vi "SETMotorOFF.vi"(8 "error in":errorcluster, 11 "PicomotorController in":refnum<class "PicomotorController.lvclass">) -> (0 "error out":errorcluster, 3 "PicomotorController out":refnum<class "PicomotorController.lvclass">)   [LabVIEW 2020, in "PicomotorController.lvclass"]
uses:
  PicomotorController.lvclass
  MCL Cmd Cluster.ctl
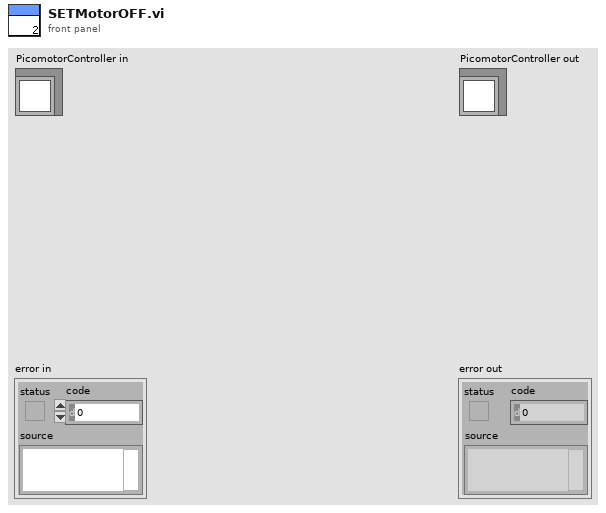
[diagram p1: front panel]
types:
  T1 = typedef "MCL Cmd Cluster.ctl" = cluster{"MCL Cmd":enum16{"User....", "DEF", "DIAG", "INI", "LOCK", "UNLOCK", "MAP", "SAV", "VER", "ACC", "CHL", "FOR", "GO", "HAL", "MOF", "MON", "MPV", "POS", "REL", "REV", "STA", "STO", "TYP", "VEL", "ABS", "SER", "NOS", "DRT", "FLI", "RLI", "FIN", "RIN", "AIN", "IN", "JOF", "JON", "OUT", "RES FINE", "RES COARSE", "02 (HEX)", "PWM", "CNT", "TMR", "HOSTNAME", "IPADDR", "IPMODE", "NETMASK", "GATEWAY", "DNSSRVR", "PASSWD", "ECHO", "MACADDR"}, "User Cmd/Numeric Argu":string, "Query/Set":enum16{"Query", "Set"}}
  T2 = typedef "VISA & TCPIP Control.ctl" = cluster{"Resource Name":refnum<visa-resource-name>, "Init VISA":bool, "Close VISA":bool, "VISA or TCP/IP":bool, "IP Address/Hostname":string}
  T3 = typedef "Pico Parameters.ctl" = cluster{"Pico Type":enum16{"Open-Loop Pico", "Close-Loop Pico", "Pico Ultra"}, "Acceleration (steps/sec^2)":string, "Velocity ( Hz)":string, "Driver":string, "Motor":string, "Channel":string, "Process Step":string}
  T4 = typedef "Error.ctl" = errorcluster
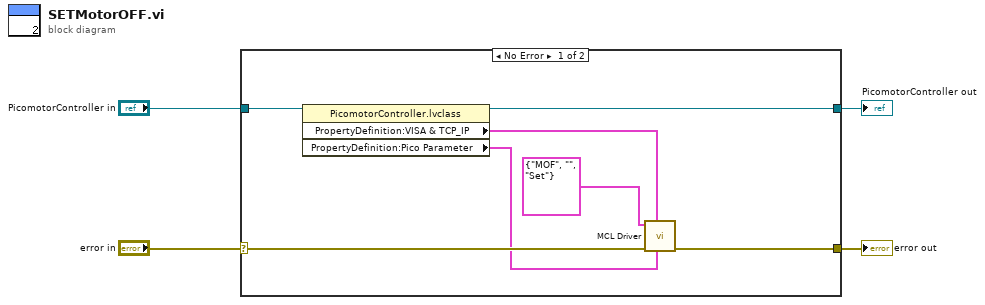
[diagram p0: block diagram]
diagram:
  n1 = case shown="No Error" "error in" {
    selector: "error in" -> [w7 w13]
    tunnel: [w6 w13] -> w3
    tunnel: [w8 w12] -> w1
    tunnel: "PicomotorController in" -> [w9 w12]
    frame No Error {
      n2 = property class="PicomotorController.lvclass"(reference=w9) -> (reference out=w8:refnum<class "PicomotorController.lvclass">, "PropertyDefinition:VISA & TCP_IP"=w11:T2, "PropertyDefinition:Pico Parameter"=w5:T3)  [unwired: 1 in, 1 out]
      n3 = call "MCL Driver.vi"("Pico Parameter"=w5, "VISA"=w11, "Error In (no error)"=w7, "MCL Command"=T1 {"MCL Cmd"=enum."MOF", "User Cmd/Numeric Argu"="", "Query/Set"=enum."Set"}) -> ("Error Out"=w6:T4)  [unwired: 3 in, 4 out]
    }
    frame Error {
    }
  }
  "error out" <- w3
  "PicomotorController out" <- w1
